vi "enter alarm_enable info in logger table.vi"(8 "error in (no error)":errorcluster, 10 "alarmenable":bool=TRUE, 11 "Shared Variable":string="LB_Energy") -> (0 "error out":errorcluster)   [LabVIEW 2013]
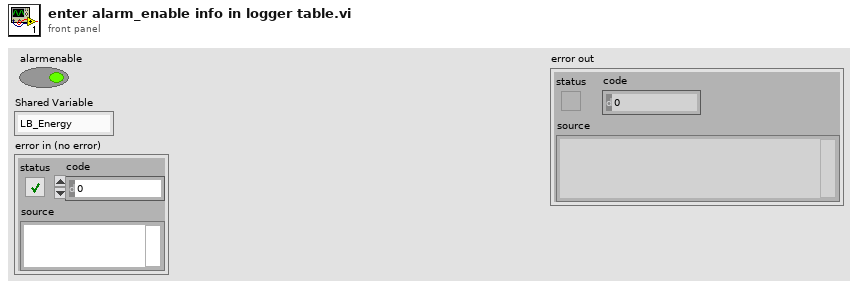
[diagram p1: front panel]
types:
  T1 = typedef "mysql_authentication.ctl" = cluster{"User":string, "Password":string, "Database":string}
  T2 = cluster{"Port":u16, "IP Address":string, "Authentication":T1}
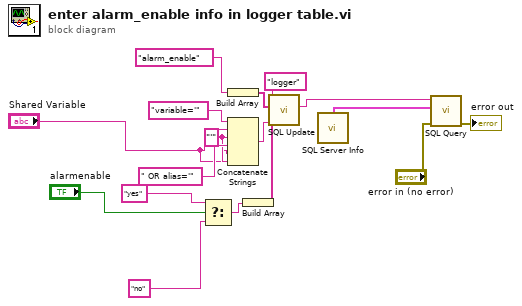
[diagram p0: block diagram]
diagram:
  w13 = "'" ("string")
  n1 = Select(t="yes", s="alarmenable", f="no") -> (s? t:f=w9:string)
  n2 = Build Array("alarm_enable") -> (w4:string[])
  n3 = Concatenate Strings("variable='", "Shared Variable", w13, " OR alias='", "Shared Variable", w13) -> (w12:string)
  n4 = Build Array(w9) -> (w8:string[])
  n5 = call "SQL Update.vi"("Where clause"=w12, "Values"=w8, "Column Names"=w4, "Table"="logger") -> ("Query String"=w7:string)  [unwired: 7 in]
  n6 = call "SQL Server Info.vi"() -> ("SQL Server Info"=w17:T2)
  n7 = call "SQL Query.vi"("error in (no error)"="error in (no error)", "SQL Server Info"=w17, "Query"=w7) -> ("error out"=→"error out":errorcluster)  [unwired: 7 in, 1 out]
